vi "Self Test.vi"(8 "error in":errorcluster, 11 "57XX in":refnum<class "57XX.lvclass">) -> (0 "error out":errorcluster, 3 "57XX out":refnum<class "57XX.lvclass">)   [LabVIEW 2019, in "57XX.lvlib" / "57XX.lvclass"]
uses:
  Library/57XX.lvclass
  builds/Instruments/PowerSupply.lvlibp/Library/PowerSupply.lvclass
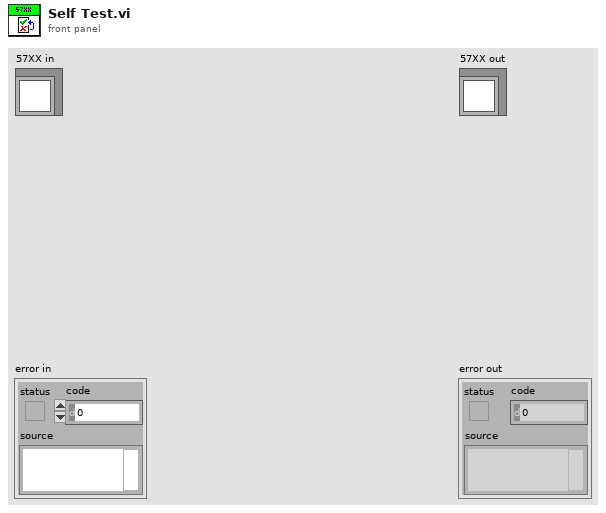
[diagram p1: front panel]
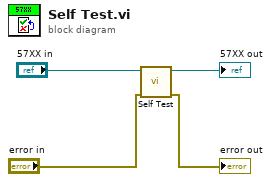
[diagram p0: block diagram]
diagram:
  n1 = call-parent "Self Test.vi"("error in"="error in", "Instruments in"="57XX in") -> ("error out"=→"error out":errorcluster, "Instruments out"=→"57XX out":refnum<class "57XX.lvclass">)  [unwired: 8 in]
